vi "uSubscriber Register.vi"(8 "error in (no error)":errorcluster, 9 "Policy (All-Topics)":refnum<class "uPolicy.lvclass">, 10 "Broker":refnum<class "uTransport_uActor.lvclass">, 11 "Subscriber's uTransport":refnum<class "uTransport.lvclass">) -> (0 "error out":errorcluster)   [LabVIEW 2023, in "uLib.lvlib" / "uClient_Subscriber.lvclass"]
uses:
  uClient_Subscriber.lvclass
  uClient/uClient.lvclass
  uTransport/uTransport/uTransport.lvclass
  uMsg/uMsg/uMsg.lvclass
  uData/uData/uData.lvclass
  uNotifyMode/uNotifyMode/uNotifyMode.lvclass
  U:/Projects/uLib/Src/uFramework/uClient/uClient.lvclass
  U:/Projects/uLib/Src/uFramework/uClient_Subscriber/uClient_Subscriber.lvclass
  uPolicy/uPolicy/uPolicy.lvclass
  uTransport/uTransport_uActor/uTransport_uActor.lvclass
  U:/Projects/uLib/Src/uFramework/uTransport_uActor/uTransport_uActor.lvclass
  U:/Projects/uLib/Src/uFramework/uTransport/uTransport.lvclass
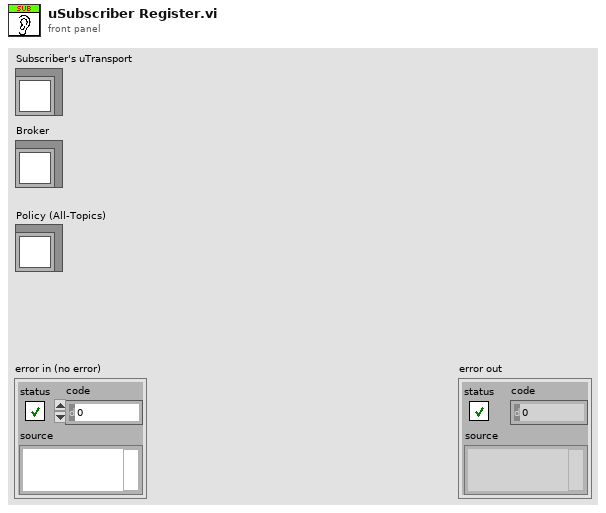
[diagram p1: front panel]
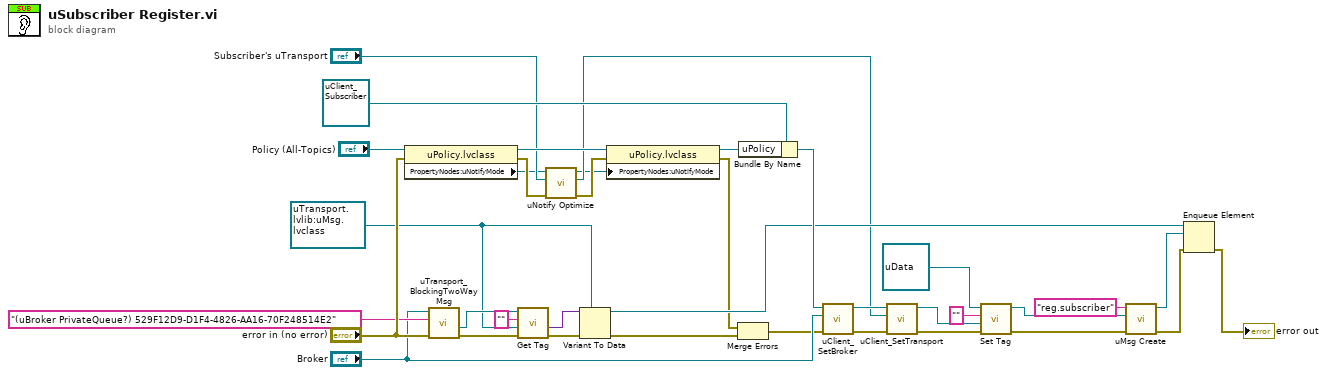
[diagram p0: block diagram]
diagram:
  w24 = refnum<queue> refnum ("brokerage queue")
  n1 = property class="uPolicy.lvclass"(reference="Policy (All-Topics)", error in="error in (no error)") -> (reference out=w9:refnum<class "uPolicy.lvclass">, error out=w34:errorcluster, "PropertyNodes:uNotifyMode"=w1:refnum<class "uNotifyMode.lvclass">)
  n2 = call "uTransport_BlockingTwoWayMsg.vi"("error in (no error)"="error in (no error)", "Command"="(uBroker PrivateQueue?) 529F12D9-D1F4-4826-AA16-70F248514E2", "uTransport in"="Broker") -> ("error out"=w28:errorcluster, "Reply"=w29:refnum<class "uData.lvclass">)  [unwired: 7 in]
  n3 = call "Get Tag.vi"("error in (no error)"=w28, "default value"=w24, "tag (case insensitive)"="", "uData in"=w29) -> ("error out"=w27:errorcluster, "value"=w25:variant)  [unwired: 4 in, 2 out]
  n4 = call "uNotify Optimize.vi"("error in (no error)"=w34, "Listener Transport in"="Subscriber's uTransport", "uNotifyMode in"=w1) -> ("error out"=w35:errorcluster, "Listener Transport out"=w3:refnum<class "uTransport.lvclass">, "uNotifyMode out"=w2:refnum<class "uNotifyMode.lvclass">)  [unwired: 6 in]
  n5 = Variant To Data(error in=w27, type=w24, Variant=w25) -> (data=w21:refnum<queue>, error out=w7:errorcluster)
  n6 = property class="uPolicy.lvclass"(reference=w9, error in=w35, "PropertyNodes:uNotifyMode"=w2) -> (reference out=w8:refnum<class "uPolicy.lvclass">, error out=w5:errorcluster)
  n7 = Merge Errors(w5, w7) -> (w6:errorcluster)
  n8 = Bundle By Name(cluster=refnum<class "uClient_Subscriber.lvclass"> refnum ("uClient_Subscriber in"), "uPolicy"=w8) -> (w30:refnum<class "uClient_Subscriber.lvclass">)
  n9 = call "uClient_SetBroker.vi"("error in (no error)"=w6, "Broker"="Broker", "uClient in"=w30) -> ("error out"=w32:errorcluster, "uClient out"=w33:refnum<class "uClient_Subscriber.lvclass">)  [unwired: 7 in]
  n10 = call "uClient_SetTransport.vi"("error in (no error)"=w32, "uTransport"=w3, "uClient in"=w33) -> ("error out"=w16:errorcluster, "uClient out"=w11:refnum<class "uClient_Subscriber.lvclass">)  [unwired: 7 in]
  n11 = call "Set Tag.vi"("error in (no error)"=w16, "Variant"=w11, "tag (case insensitive)"="", "uData in"=refnum<class "uData.lvclass"> refnum) -> ("error out"=w15:errorcluster, "uData out"=w14:refnum<class "uData.lvclass">)  [unwired: 5 in, 1 out]
  n12 = call "uMsg Create.vi"("error in (no error)"=w15, "Payload"=w14, "CMD"="reg.subscriber") -> ("error out"=w18:errorcluster, "uMsg out"=w19:refnum<class "uMsg.lvclass">)  [unwired: 7 in]
  n13 = Enqueue Element(queue=w21, element=w19, error in (no error)=w18) -> (error out=→"error out":errorcluster)  [unwired: 1 in, 2 out]
